vi "Cal IC (VIRef).vi"(8 "error in (no error)":errorcluster, 10 "IC in":variant, 11 "Domain_Evolut_1D in":refnum<class "NI_Domain_Evolut_1D.lvclass">) -> (0 "error out":errorcluster, 2 "IC out":variant, 3 "Domain_Evolut_1D out":refnum<class "NI_Domain_Evolut_1D.lvclass">)   [LabVIEW 2020, in "NI_PDE.lvlib" / "NI_Domain_Evolut_1D.lvclass"]
uses:
  <vilib>/gmath/pde.llb/DomainClass/Domain_Evolut_1D/NI_Domain_Evolut_1D.lvclass
  <vilib>/gmath/pde.llb/ICClass/IC_1D_VIRef/IC Data.ctl
  <vilib>/gmath/pde.llb/Common/PDE_IC Type.ctl
  <vilib>/gmath/pde.llb/ICClass/IC_1D_Numeric/IC Data.ctl
  <vilib>/gmath/pde.llb/DomainClass/Domain_Evolut_1D/NI_Domain_Evolut_1D.lvclass/NI_Domain_Evolut_1D.ctl
  <vilib>/Analysis/1siggen.llb/Ramp Pattern by Samples.vi
  <vilib>/gmath/NI_PDE.lvlib
  <vilib>/gmath/pde.llb/ICClass/IC_1D_VIRef/NI_IC_1D_VIRef.lvclass
  <vilib>/gmath/pde.llb/ICClass/IC_1D_Numeric/NI_IC_1D_Numeric.lvclass
  <vilib>/Analysis/NI_AALBase.lvlib
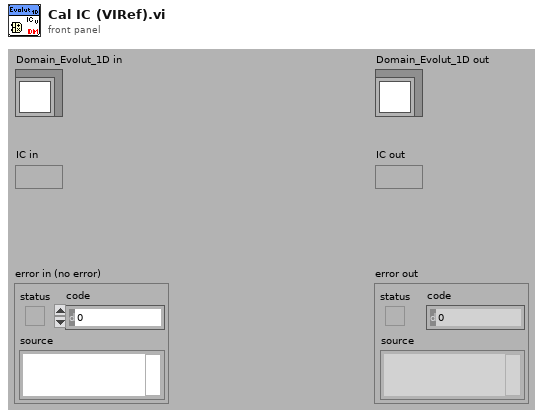
[diagram p1: front panel]
types:
  T1 = typedef "NI_PDE.lvlib/NI_IC_1D_Numeric.lvclass/IC Data.ctl" = cluster{"type":T2, "H":dbl[]}
  T2 = typedef "NI_PDE.lvlib/PDE_IC Type.ctl" = i32
  T3 = typedef "NI_PDE.lvlib/NI_IC_1D_VIRef.lvclass/IC Data.ctl" = cluster{"type":T2, "H":refnum<vi>, "data":variant}
  T4 = cluster{"initial t":dbl, "final t":dbl, "# of t-points":i32}
  T5 = cluster{"start x":dbl, "end x":dbl, "# of x-points":i32}
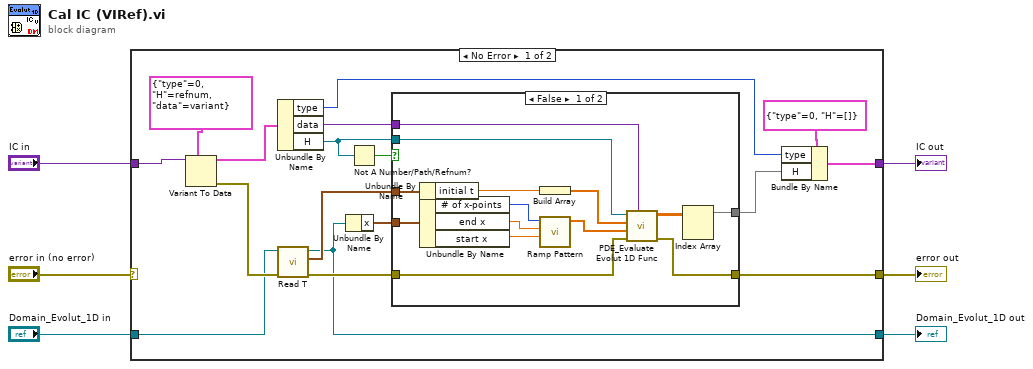
[diagram p0: block diagram]
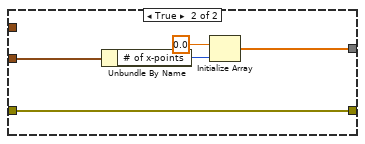
[diagram p2: hidden frame]
diagram:
  n1 = case shown="No Error" "error in (no error)" {
    selector: "error in (no error)" -> [_ w45]
    tunnel: "Domain_Evolut_1D in" -> [w8 w44]
    tunnel: [w7 w44] -> w6
    tunnel: [w13 w45] -> w5
    tunnel: [w15 w43] -> w2
    tunnel: "IC in" -> [w14 w43]
    frame No Error {
      n2 = Variant To Data(type=T3 {"type"=0, "H"=refnum, "data"=variant} ("IC data"), Variant=w14) -> (data=w19:T3, error out=w9:errorcluster)  [unwired: 1 in]
      n3 = Unbundle By Name(w19) -> ("type"=w17:T2, "data"=w21:variant, "H"=w22:refnum<vi>)
      n4 = call-dynamic "Read T.vi"("error in (no error)"=w9, "Domain_Evolut.lvclass in"=w8) -> ("error out"=w10:errorcluster, "t"=w12:T4, "Domain_Evolut.lvclass out"=w7:refnum<class "NI_Domain_Evolut_1D.lvclass">)  [unwired: 7 out]
      n5 = Unbundle By Name(w7) -> ("x"=w11:T5)
      n6 = Not A Number/Path/Refnum?(number/path/refnum=w22) -> (NaN/Path/Refnum?=w23:bool)
      n7 = case shown="False" w23 {
        tunnel: [w32 w42] -> w16
        tunnel: w12 -> [w37 _]
        tunnel: w10 -> [w31 w40]
        tunnel: [w36 w40] -> w13
        tunnel: w22 -> [w35 _]
        tunnel: w21 -> [w34 _]
        tunnel: w11 -> [w30 w38]
        frame False {
          n8 = Unbundle By Name(w37) -> ("initial t"=w29:dbl)
          n9 = Unbundle By Name(w30) -> ("# of x-points"=w25:i32, "end x"=w27:dbl, "start x"=w26:dbl)
          n10 = Build Array(w29) -> (w28:dbl[])
          n11 = call-poly <vilib>:"Ramp Pattern.vi"("start"=w26, "end"=w27, "samples"=w25) -> ("Ramp Pattern"=w24:dbl[])  [unwired: 7 in, 1 out]
          n12 = call <vilib>:"PDE_Evaluate Evolut 1D Func.vi"("data"=w34, "error in (no error)"=w31, "X"=w24, "T"=w28, "VIRef"=w35) -> ("error out"=w36:errorcluster, "F(t, x)"=w33:dbl[][])  [unwired: 5 out]
          n13 = Index Array(array=w33) -> (element=w32:dbl[])  [unwired: 2 in]
        }
        frame True {
          n14 = Unbundle By Name(w38) -> ("# of x-points"=w39:i32)
          n15 = Initialize Array(0.0 ("element"), w39) -> (w42:dbl[])
        }
      }
      n16 = Bundle By Name(cluster=T1 {"type"=0, "H"=[]} ("IC data"), "type"=w17, "H"=w16) -> (w15:T1)
    }
    frame Error {
    }
  }
  "Domain_Evolut_1D out" <- w6
  "error out" <- w5
  "IC out" <- w2
